vi "Build Array Histogram.vi"(4 "Weights":dbl[](array[numeric]), 5 "Normalized Weighted Histogram":bool, 6 "Data Type (Plot Y Axis)":T4, 7 "Graph Caption (or Label) Text":string, 8 "error in (no error)":errorcluster, 9 "Histogram Options":T1 {"Max Histogram Size" format="%.0e"}, 10 "Plot/Dataset Name":string, 11 "Array":dbl[](array[numeric])) -> (0 "error out":errorcluster, 1 "Message":string, 3 "Data Statistics":dbl[](array[numeric]))   [LabVIEW 2021, in "Histogram Window.lvlib"]
uses:
  Histogram Window.lvlib
  Source Data Type.ctl
  Linear Histogram Options.ctl
  Histogram Bin Option.ctl
  Histogram Bin Position.ctl
  Plot Histogram.ctl
  Graphs/Plot Style 3.ctl
  Histogram Data Statistics.ctl
  Histogram Window Q Element v2.ctl
  Histogram Window Q Action v2.ctl
  1d04790c-9f2d-4c42-9419-74125c4f92e4.vi
  1d04790c-9f2d-4c42-9419-74125c4f92e4.vi/e021cd17-e000-4244-b7f4-ec50548bdfcb.vi
  1d04790c-9f2d-4c42-9419-74125c4f92e4.vi/b1828c6e-eb0a-43e9-a724-8b596c52e435.vi
  1d04790c-9f2d-4c42-9419-74125c4f92e4.vi/7a6138ed-c001-4311-b538-9ba42ae7c7b1.vi
  1d04790c-9f2d-4c42-9419-74125c4f92e4.vi/52c6b4fa-501b-4af0-803b-8bab516ca5d3.vi
  1d04790c-9f2d-4c42-9419-74125c4f92e4.vi/d7237e10-35ab-4bcb-a0c6-4883c3f4c990.vi
  1d04790c-9f2d-4c42-9419-74125c4f92e4.vi/5fb5dd96-3b97-4592-ba56-58181c8e7105.vi
  1d04790c-9f2d-4c42-9419-74125c4f92e4.vi/8e13a849-a393-4484-9968-4af7b25c38d7.vi
  Histogram Window.vi
  <userlib>/_OpenG.lib/array/array.llb/Filter 1D Array (DBL)__ogtk.vi
  <userlib>/_OpenG.lib/array/array.llb/Delete Elements from 1D Array (DBL)__ogtk.vi
  <vilib>/Analysis/baseanly.llb/Unimode.vi
  Time/High Resolution Timing.vi
  <vilib>/Utility/error.llb/Error Cluster From Error Code.vi
  Graphs/Graphs.lvlib
  Utilities/Utilities.lvlib
  <vilib>/Analysis/NI_AALBase.lvlib
  <userlib>/_OpenG.lib/array/array.llb/openg_array.lvlib
  Math/Math.lvlib
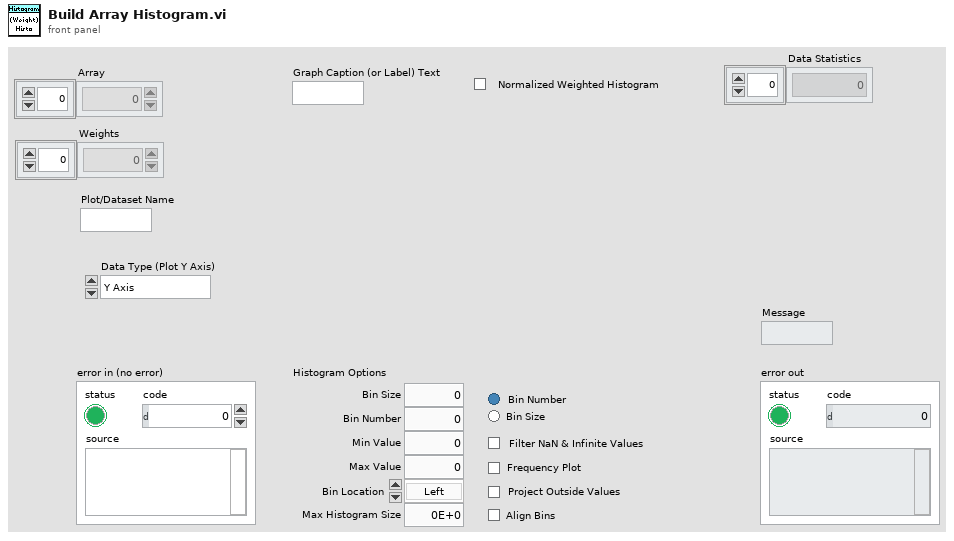
[diagram p1: front panel]
types:
  T1 = typedef "Histogram Window.lvlib/Linear Histogram Options.ctl" = cluster{"Bin Size":dbl, "Bin Number":i32, "Bin Option":T2, "Min Value":dbl, "Max Value":dbl, "Filter NaN & Infinite Values":bool, "Frequency Plot":bool, "Align Bins":bool, "Bin Location":T3, "Project Outside Values":bool, "Max Histogram Size":i32}
  T2 = typedef "Histogram Window.lvlib/Histogram Bin Option.ctl" = enum32{"Bin Number", "Bin Size"}
  T3 = typedef "Histogram Window.lvlib/Histogram Bin Position.ctl" = enum16{"Left", "Center", "Right"}
  T4 = typedef "Histogram Window.lvlib/Source Data Type.ctl" = enum16{"Y Axis", "X Axis", "Single Array"}
  T5 = typedef "Graphs.lvlib/Plot Style 3.ctl" = cluster{"Plot Style":enum16{"unchanged", "Line", "Symbol", "Line + Symbol", "Histogram", "Histogram + Symbol"}, "Histogram Type":enum16{"unchanged", "Left Bound", "Center", "Right Bound"}, "Line Tickness":enum16{"unchanged", "Thin", "1 pixel", "2 pixel", "3 pixel", "4 pixel", "5 pixel"}, "Line Style":enum16{"unchanged", "Plain", "Long Dash", "Short Dash", "Long-Short Dash", "Long-Short-Short Dash"}, "Point Style":enum16{"unchanged", "None", "Empty Circle", "Filled Circle", "Thick Circle", "Dotted Circle", "Empty Square", "Filled Square", "Thick Square", "Dotted Square", "Small Filled Square", "Dot", "Cross", "Tiny Cross", "Large X", "Small x", "Diamond", "Small Empty Square"}, "Line Color":u32, "Point Color":u32, "Anti-aliased":bool, "Line Color Chooser":enum16{"unchanged", "Color Box", "Color List"}, "Point Color Chooser":enum16{"unchanged", "Color Box", "Color List"}, "Line Color List":string, "Point Color List":string}
  T6 = typedef "Histogram Window.lvlib/Histogram Window Q Element v2.ctl" = cluster{"Histogram Window Q Action":T7, "Data":variant}
  T7 = typedef "Histogram Window.lvlib/Histogram Window Q Action v2.ctl" = enum16{"Idle", "Initialization", "Generic XY Graph Event", "Add Histogram", "Delete Plot", "Delete Selected Plots", "Clear Graph", "Change Bin Size", "Invert Histogram", "Update Graph", "Plot Fit", "Export XYGraph to Notebook", "Set Last Cursor Style", "Quit"}
  T8 = typedef "Histogram Window.lvlib/Histogram Data Statistics.ctl" = cluster{"mean":dbl, "standard deviation":dbl, "variance":dbl, "rms value":dbl, "median":dbl, "mode":dbl, "max Value":dbl, "min Value":dbl, "# elements  ":dbl}
  T9 = typedef "Histogram Window.lvlib/Plot Histogram.ctl" = cluster{"Plot Name":string, "Histogram":cluster{"Axis":dbl[], "Histogram":dbl[]}, "Plot Style":T5}
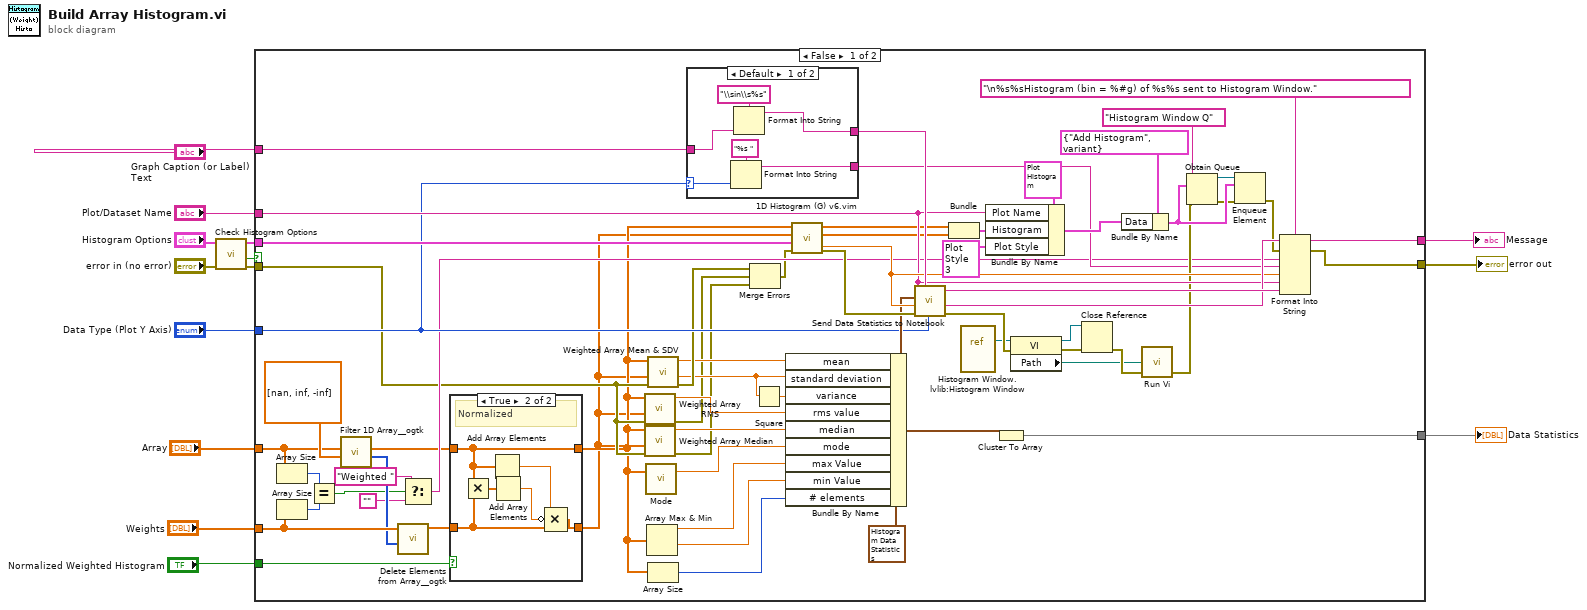
[diagram p0: block diagram]
diagram:
  n1 = call "Check Histogram Options.vi"("error in (no error)"="error in (no error)", "Histogram Options in"="Histogram Options") -> ("error out"=w4:errorcluster, "Cancelled?"=w3:bool, "Histogram Options out"=w5:T1)  [unwired: 7 in]
  n2 = case shown="False" w3 {
    tunnel: "Data Type (Plot Y Axis)" -> [w39 _]
    tunnel: "Graph Caption (or Label) Text" -> [w38 _]
    tunnel: "Plot/Dataset Name" -> [w68 _]
    tunnel: [w66 _] -> w11
    tunnel: [w65 w92] -> w10
    tunnel: "Array" -> [w36 _]
    tunnel: [w62 _] -> w8
    tunnel: w5 -> [w40 _]
    tunnel: w4 -> [w21 w92]
    tunnel: "Weights" -> [w33 _]
    tunnel: "Normalized Weighted Histogram" -> [w19 _]
    frame False {
      n3 = Array Size(array=w36) -> (size(s)=w35:i32)
      n4 = Array Size(array=w33) -> (size(s)=w34:i32)
      n5 = Equal?(x=w35, y=w34) -> (x = y?=w27:bool)
      n6 = call-poly <userlib>:"Filter 1D Array__ogtk.vi"("items to filter"=dbl[] [nan, inf, -inf] ("Element(s) to Remove"), "array"=w36) -> ("filtered item indices"=w32:i32[], "filtered array"=w18:dbl[])  [unwired: 4 in]
      n7 = call-poly <userlib>:"Delete Elements from Array__ogtk.vi"("indices"=w32, "array"=w33) -> ("array w/ subset deleted"=w16:dbl[])  [unwired: 8 in, 1 out]
      n8 = Select(t="Weighted " ("input 1"), s=w27, f="") -> (s? t:f=w24:string)
      n9 = case shown="True" w19 {
        tunnel: w18 -> [w79 w84]
        tunnel: [w79 w84] -> w17
        tunnel: w16 -> [w78 w83]
        tunnel: [w78 w80] -> w15
        frame False {
        }
        frame True {
          # "Normalized"
          n10 = Multiply(x=w84, y=w83) -> (x*y=w85:dbl[])
          n11 = Add Array Elements(numeric array=w84) -> (sum=w82:dbl)
          n12 = Add Array Elements(numeric array=w85) -> (sum=w81:dbl)
          n13 = Compound Arithmetic op=MULTIPLY(w82, invert w81, w83) -> (w80:dbl[])
        }
      }
      n14 = call "Weighted Array RMS.vi"("Error In"=w21, "Weight Array"=w15, "X Array"=w17) -> ("Error Out"=w22:errorcluster, "RMS"=w51:dbl)  [unwired: 6 in, 1 out]
      n15 = call "Weighted Array Median.vi"("Error In"=w21, "Weight Array"=w15, "X Array"=w17) -> ("Error Out"=w20:errorcluster, "Median"=w52:dbl)  [unwired: 6 in, 1 out]
      n16 = call-poly <vilib>:"Mode.vi"("X"=w17) -> ("mode"=w53:dbl)  [unwired: 1 in, 1 out]
      n17 = Array Max & Min(array=w17) -> (max value=w54:dbl, min value=w55:dbl)  [unwired: 2 out]
      n18 = call "Weighted Array Mean & SDV.vi"("Error In"=w21, "Weight Array"=w15, "Array"=w17) -> ("Error Out"=w31:errorcluster, "SDV (weighted)"=w29:dbl, "Average Value (weighted)"=w30:dbl)  [unwired: 3 in, 3 out]
      n19 = Array Size(array=w17) -> (size(s)=w56:i32)
      n20 = case shown="Default" w39 {
        selector: w39 -> [w88 _]
        tunnel: [w90 _] -> w77
        tunnel: w38 -> [w89 _]
        tunnel: [w87 _] -> w37
        frame Default {
          n21 = Format Into String(format string="%s ", w88) -> (resulting string=w87:string)  [unwired: 2 in, 1 out]
          n22 = Format Into String(format string="\\sin\\s%s", w89) -> (resulting string=w90:string)  [unwired: 2 in, 1 out]
        }
        frame "Single Array" {
          # "if not from a plot, the \"source graph\" and \"axis\" are meaningless"
        }
      }
      n23 = Merge Errors(w31, w22, w20) -> (w23:errorcluster)
      n24 = Square(x=w29) -> (x^2=w28:dbl)
      n25 = Bundle By Name(cluster=T8 {"mean"=0.0, "standard deviation"=0.0, "variance"=0.0, "rms value"=0.0, "median"=0.0, "mode"=0.0, "max Value"=0.0, "min Value"=0.0, "# elements  "=0.0} ("Data Statistics"), "mean"=w30, "standard deviation"=w29, "variance"=w28, "rms value"=w51, "median"=w52, "mode"=w53, "max Value"=w54, "min Value"=w55, "# elements"=w56) -> (w61:T8)
      n26 = call "1D Histogram (G) v6.vim"("Error In"=w23, "Histogram Options"=w40, "Weights"=w15, "Array"=w17) -> ("Error Out"=w75:errorcluster, "Histogram"=w47:dbl[], "Axis"=w48:dbl[], "Actual Bin Size"=w74:dbl)  [unwired: 1 in, 3 out]
      n27 = call "Send Data Statistics to Notebook.vi"("Source Data Type (Plot Y Axis)"=w39, "Graph Caption"=w77, "Error In"=w75, "Bin"=w74, "Data Statistics"=w61, "Plot/Dataset Name"=w68) -> ("Error Out"=w60:errorcluster, "Message"=w76:string)  [unwired: 4 in]
      n28 = Bundle("Axis"=w48, "Histogram"=w47) -> (w42:cluster{"Axis":dbl[], "Histogram":dbl[]})  [unwired: 1 in]
      n29 = vi-ref "Histogram Window.lvlib:Histogram Window.vi"() -> (w57:refnum<vi>)
      n30 = Bundle By Name(cluster=T9 {"Plot Name"="", "Histogram"={"Axis"=[], "Histogram"=[]}, "Plot Style"={"Plot Style"=enum."Histogram + Symbol", "Histogram Type"=enum."Right Bound", "Line Tickness"=enum."unchanged", "Line Style"=enum."unchanged", "Point Style"=enum."unchanged", "Line Color"=0, "Point Color"=0, "Anti-aliased"=FALSE, "Line Color Chooser"=enum."unchanged", "Point Color Chooser"=enum."unchanged", "Line Color List"="", "Point Color List"=""}} ("output cluster"), "Plot Name"=w68, "Histogram"=w42, "Plot Style"=T5 {"Plot Style"=enum."Histogram", "Histogram Type"=enum."Left Bound", "Line Tickness"=enum."1 pixel", "Line Style"=enum."Plain", "Point Style"=enum."None", "Line Color"=0, "Point Color"=0, "Anti-aliased"=TRUE, "Line Color Chooser"=enum."Color Box", "Point Color Chooser"=enum."unchanged", "Line Color List"="", "Point Color List"=""}) -> (w46:T9)
      n31 = Cluster To Array(cluster=w61) -> (array=w62:dbl[])
      n32 = property class="VI"(reference=w57, error in=w60) -> (reference out=w58:refnum<vi>, error out=w72:errorcluster, "Path"=w59:path)
      n33 = Close Reference(reference=w58, error in (no error)=w72) -> (error out=w73:errorcluster)
      n34 = Bundle By Name(cluster=T6 {"Histogram Window Q Action"=enum."Add Histogram", "Data"=variant} ("ALEX TT Histogram Q Element"), "Data"=w46) -> (w70:T6)
      n35 = call "Run Vi.vi"("VI Path"=w59, "error in (no error)"=w73) -> ("error out"=w49:errorcluster)  [unwired: 6 in, 1 out]
      n36 = Obtain Queue(name (unnamed)="Histogram Window Q", element data type=w70, error in (no error)=w49) -> (queue out=w43:refnum<queue>, error out=w45:errorcluster)  [unwired: 2 in, 1 out]
      n37 = Enqueue Element(queue=w43, element=w70, error in (no error)=w45) -> (error out=w64:errorcluster)  [unwired: 1 in, 2 out]
      n38 = Format Into String(format string="\n%s%sHistogram (bin = %#g) of %s%s sent to Histogram Window.", initial string=w76, error in=w64, w24, w37, w74, w68, w77) -> (resulting string=w66:string, error out=w65:errorcluster)
    }
    frame True {
    }
  }
  "Message" <- w11
  "error out" <- w10
  "Data Statistics" <- w8
